vi "Remove Subscriber.vi"(8 "error in (no error)":errorcluster, 9 "Unsubscription Object":refnum<class>, 10 "Unsubscriber Enqueuer":refnum<class "Message Enqueuer.lvclass">, 11 "Subsciptions in":T1[](array[typedef])) -> (0 "error out":errorcluster, 3 "Subsciptions out":T1[](array[typedef]))   [LabVIEW 2020, in "Publisher.lvlib" / "Publisher.lvclass"]
doc: "Remove the 'Unsubscriber Enqueuer' from the 'Subscriptions' using the 'Subscription string'."
uses:
  Publisher.lvclass
  PPL/HDH.Actor Framework.Core.Actor.lvlibp/1abvi3w/vi.lib/ActorFramework/Message Enqueuer/Message Enqueuer.lvclass
  Controls/Ctl_Subscription Element.ctl
  PPL/HDH.Actor Framework.Core.Utility.lvlibp
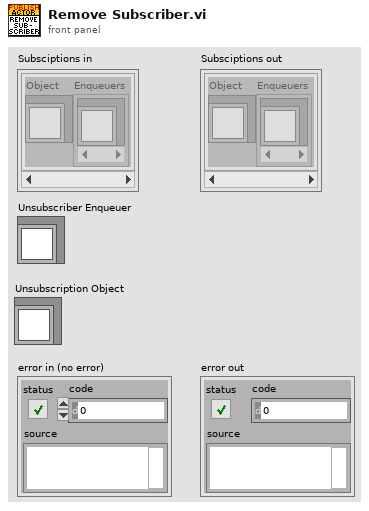
[diagram p1: front panel]
types:
  T1 = typedef "Publisher.lvlib/Publisher.lvclass/Ctl_Subscription Element.ctl" = cluster{"Object":refnum<class>, "Enqueuers":refnum<class "Message Enqueuer.lvclass">[]}
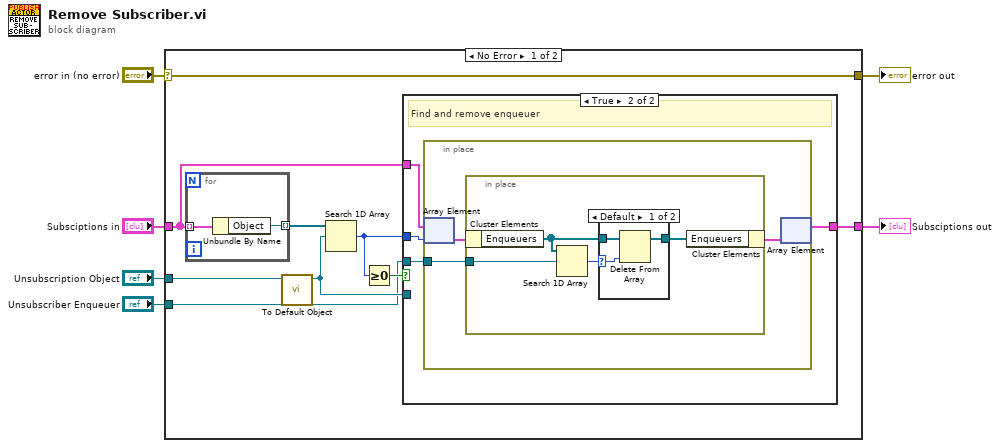
[diagram p0: block diagram]
diagram:
  n1 = case shown="No Error" "error in (no error)" {
    selector: "error in (no error)" -> [w7 w35]
    tunnel: "Unsubscription Object" -> [w15 _]
    tunnel: "Subsciptions in" -> [w12 w34]
    tunnel: "Unsubscriber Enqueuer" -> [w10 _]
    tunnel: [w9 w34] -> w3
    tunnel: [w7 w35] -> w2
    frame No Error {
      n2 = for {
        tunnel: w12 -> [w33] mode=indexing
        tunnel: [w32] -> w14 mode=indexing
        n3 = Unbundle By Name(w33) -> ("Object"=w32:refnum<class>)
      }
      n4 = call "To Default Object.vi"("Object in"=w15) -> ("Default out"=w11:refnum<class>)  [unwired: 10 in]
      n5 = Search 1D Array(1D array=w14, element=w11) -> (index of element=w8:i32)  [unwired: 1 in]
      n6 = Greater Or Equal To 0?(x=w8) -> (x >= 0?=w13:bool)
      n7 = case shown="True" w13 {
        tunnel: w12 -> [w16 w20]
        tunnel: w11 -> [_ _]
        tunnel: w10 -> [_ w18]
        tunnel: [w16 w19] -> w9
        tunnel: w8 -> [_ w17]
        frame False {
          # "No subscription - Do nothing"
        }
        frame True {
          # "Find and remove enqueuer"
          n8 = in-place {
            in-place-border: w18 -> [w22]
            n9 = in-place-array #1(w20, w17) -> (w23:T1)
            n10 = in-place {
              in-place-border: w22 -> [w27]
              n11 = in-place-cluster #2(w23) -> ("Enqueuers"=w24:refnum<class "Message Enqueuer.lvclass">[])
              n12 = Search 1D Array(1D array=w24, element=w27) -> (index of element=w26:i32)  [unwired: 1 in]
              n13 = case shown="Default" w26 {
                selector: w26 -> [w29 _]
                tunnel: [w28 w31] -> w25
                tunnel: w24 -> [w30 w31]
                frame Default {
                  n14 = Delete From Array(array=w30, index=w29) -> (array with subset deleted=w28:refnum<class "Message Enqueuer.lvclass">[])  [unwired: 1 in, 1 out]
                }
                frame -1 {
                }
              }
              n15 = in-place-cluster #2("Enqueuers"=w25) -> (w21:T1)
            }
            n16 = in-place-array #1(w21) -> (w19:T1[])  [unwired: 1 out]
          }
        }
      }
    }
    frame Error {
    }
  }
  "error out" <- w2
  "Subsciptions out" <- w3
